vi "UpdateImages.vi"(0 "image size (pixel)":cluster{u32, u32, u32}, 1 "1nd axis":u16, 2 "2nd axis":u16, 3 "show image":bool, 4 "retrace":bool) -> ()   [LabVIEW 2009]
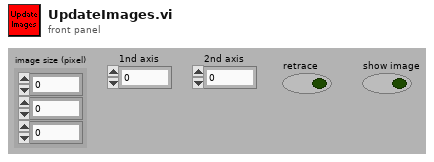
[diagram p1: front panel]
types:
  T1 = typedef "DAQLinescanVisualization.ctt" = cluster{"Threshold":u32, "Trace Window #":u32, "IMAQ Trace":T2, "Retrace Window #":u32, "IMAQ Retrace":T2}
  T2 = typedef "IMAQ Image.ctl" = refnum<image>
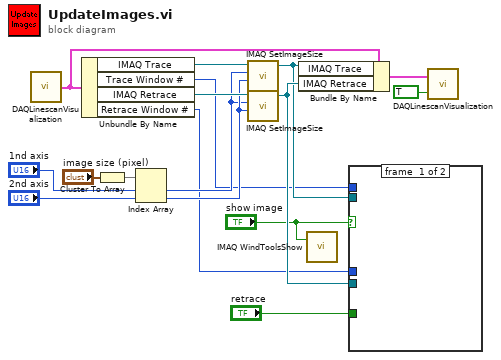
[diagram p0: block diagram]
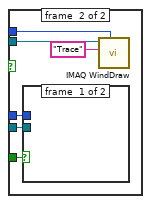
[diagram p2: hidden frame]
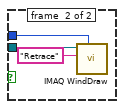
[diagram p3: hidden frame]
diagram:
  n1 = call "DAQLinescanVisualization.vi"() -> ("Visualization (output)"=w4:T1)  [unwired: 2 in]
  n2 = Unbundle By Name(w4) -> ("IMAQ Trace"=w11:T2, "Trace Window #"=w6:u32, "IMAQ Retrace"=w13:T2, "Retrace Window #"=w7:u32)
  n3 = Cluster To Array(cluster="image size (pixel)") -> (array=w5:u32[])
  n4 = Index Array(array=w5, index #1="1nd axis", index #2="2nd axis") -> (element #1=w8:u32, element #2=w9:u32)
  n5 = call "IMAQ SetImageSize"("Y Resolution"=w9, "X Resolution"=w8, "Image"=w11) -> ("Image Out"=w12:T2)  [unwired: 2 in, 1 out]
  n6 = call "IMAQ SetImageSize"("Y Resolution"=w9, "X Resolution"=w8, "Image"=w13) -> ("Image Out"=w14:T2)  [unwired: 2 in, 1 out]
  n7 = Bundle By Name(cluster=w4, "IMAQ Trace"=w12, "IMAQ Retrace"=w14) -> (w3:T1)
  n8 = call "IMAQ WindToolsShow"("Hide/Show (Show)"="show image") -> ()  [unwired: 4 in, 2 out]
  n9 = case shown="True" "show image" {
    tunnel: w6 -> [_ w22]
    tunnel: w12 -> [_ w21]
    tunnel: w7 -> [_ w20]
    tunnel: w14 -> [_ w19]
    tunnel: "retrace" -> [_ w18]
    frame #0 {
    }
    frame #1 {
      n10 = case shown="True" w18 {
        tunnel: w20 -> [_ w25]
        tunnel: w19 -> [_ w24]
        frame #0 {
        }
        frame #1 {
          n11 = call "IMAQ WindDraw"("Window Number (0...15)"=w25, "Title"="Retrace" ("Image Name"), "Image"=w24) -> ()  [unwired: 7 in, 2 out]
        }
      }
      n12 = call "IMAQ WindDraw"("Window Number (0...15)"=w22, "Title"="Trace" ("Image Name"), "Image"=w21) -> ()  [unwired: 7 in, 2 out]
    }
  }
  n13 = call "DAQLinescanVisualization.vi"("Get/Set"=TRUE, "Visualization (input)"=w3) -> ()  [unwired: 1 out]
